vi "WRP Get Acquired Data Vector Int32.vi"(8 "error in (no error)":errorcluster, 9 "size":i32, 10 "index":i32, 11 "parameter":string) -> (0 "error out":errorcluster, 1 "size out":i32, 2 "function return":i32, 3 "data":i32[](array[numeric]))   [LabVIEW 2018, in "SesWrapper.lvlib"]
doc: "int STDCALL WRP_GetAcquiredDataVectorInt32(const String parameter, int index, VectorInt32 *data, int *size);"
uses:
  SesWrapper.lvlib
  build/Debug/SESWrapper.dll
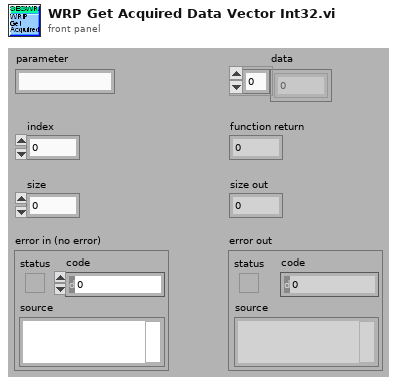
[diagram p1: front panel]
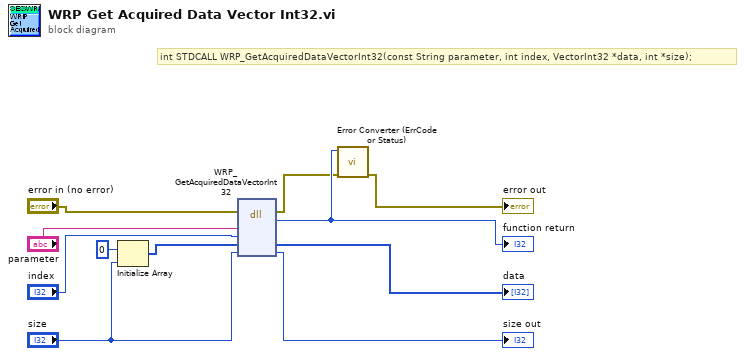
[diagram p0: block diagram]
diagram:
  # "int STDCALL WRP_GetAcquiredDataVectorInt32(const String parameter, int index, VectorInt32 *data, int *size);"
  n1 = Initialize Array(0 ("element"), "size") -> (w8:i32[])
  n2 = dll-call lib="C:/Development/svn/seswrapper-lib/build/Debug/SESWrapper.*" fn="WRP_GetAcquiredDataVectorInt32"(error in="error in (no error)", "parameter"="parameter", "index"="index", "data"=w8, "size"="size") -> (error out=w2:errorcluster, w11:i32, "data"=→"data":i32[], "size"=→"size out":i32)  [unwired: 4 in, 1 out]
  "function return" <- w11
  n3 = call "Error Converter (ErrCode or Status).vi"("error in (no error)"=w2, "error code"=w11) -> ("error out"=→"error out":errorcluster)  [unwired: 9 in]
